vi "read TDMS file -- wavefront -- V1.vi"(6 "Data type":waveform(dbl), 7 "tdms file in":refnum<k34>, 8 "error in":errorcluster, 9 "Data File Type":T2(ring), 10 "Data window":T1={"Start"=0, "Length"=500000, "Channel numbers"=[0], "Channel name"="Vpick", "Group name"="p"}, 11 "Input file path":path) -> (0 "error out":errorcluster, 1 "1st channel length":u64=433333, 2 "Data out":waveform(dbl), 3 "Actual input file path":path, 5 "tdms file out":refnum<k34>)   [LabVIEW 2021]
uses:
  tdo - old/Data window.ctl
panel:
  # "OR"
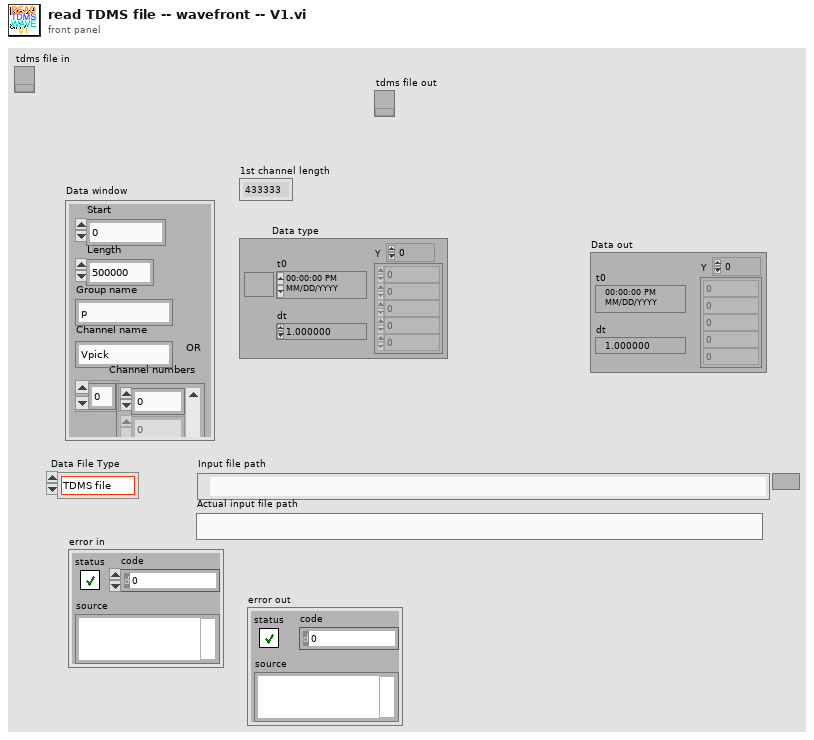
[diagram p1: front panel]
types:
  T1 = typedef "Data window.ctl" = cluster{"Start":i64, "Length":i64, "Channel numbers":i64[], "Channel name":string, "Group name":string}
  T2 = enum16{"TDMS file", "Tektronics ISF", "BinF file", "ASCII File", "BinH File", "BinW File", "BINARY File"}
  T3 = enum16{"open", "open or create", "create or replace", "create", "open (read-only)"}
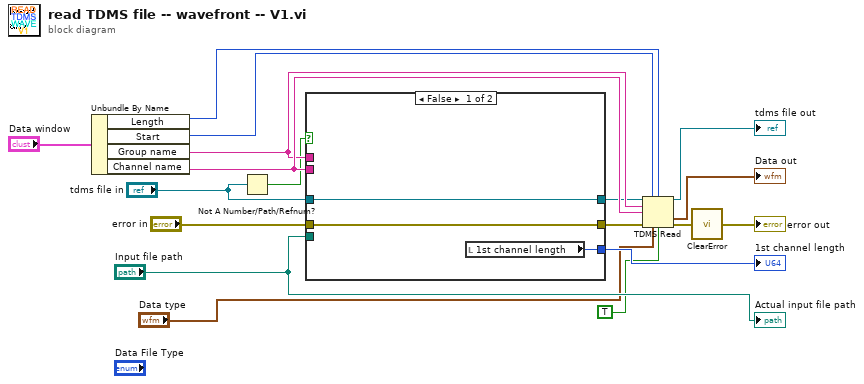
[diagram p0: block diagram]
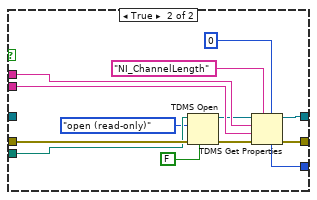
[diagram p2: hidden frame]
diagram:
  n1 = Unbundle By Name("Data window") -> ("Length"=w16:i64, "Start"=w6:i64, "Group name"=w13:string, "Channel name"=w15:string)
  n2 = Not A Number/Path/Refnum?(number/path/refnum="tdms file in") -> (NaN/Path/Refnum?=w3:bool)
  n3 = case shown="False" w3 {
    tunnel: "error in" -> [w20 w34]
    tunnel: [w21 w23] -> w5
    tunnel: [w20 w28] -> w4
    tunnel: "Input file path" -> [_ w33]
    tunnel: "tdms file in" -> [w21 _]
    tunnel: [w19 w27] -> w14
    tunnel: w15 -> [_ w26]
    tunnel: w13 -> [_ w25]
    frame False {
      n4 = local read "1st channel length"() -> (w19:u64)
    }
    frame True {
      n5 = TDMS Open(6:FALSE ("disable buffering (T)"), 8:w34, 10:T3."open (read-only)" ("operation (0:open)"), 11:w33) -> (0:w29:errorcluster, 3:w24:refnum<k34>)  [unwired: 3 in]
      n6 = TDMS Get Properties(5:u64 0, 7:"NI_ChannelLength" ("property name"), 8:w29, 9:w26, 10:w25, 11:w24) -> (0:w28:errorcluster, 3:w23:refnum<k34>, 4:w27:u64)  [unwired: 3 out]
    }
  }
  "1st channel length" <- w14
  n7 = TDMS Read(0:w5, 1:w6, 2:w16, 5:w13, 7:w15, 11:w4, 12:"Data type", 13:TRUE ("return channels in file order? (F)")) -> (4:→"tdms file out":refnum<k34>, 10:→"Data out":waveform(dbl), 15:w2:errorcluster)  [unwired: 3 out]
  n8 = call <vilib>:"ClearError.vi"("error in (no error)"=w2) -> ("error out"=→"error out":errorcluster)
  "Actual input file path" <- "Input file path"
